vi "RM.getAllDeviceInfo.vi"(8 "error in":errorcluster, 11 "Item Ref in":T2 format="%.0x") -> (0 "error out":errorcluster, 2 "deviceInfo array":T1[](array[typedef]) {"cd node ref" format="%.0x"}, 3 "Item Ref out":T2 format="%.0x")   [LabVIEW 2016, in "FPGA Resource Manager.lvlib"]
uses:
  FPGA Resource Manager.lvlib
  <vilib>/NI Veristand/Custom Device API/Custom Device Item Ref.ctl
  RM.serverInfo.ctl
  RM.Globals.vi
  <vilib>/NI Veristand/Custom Device API/Get Item Property (Variant).vi
  <vilib>/NI Veristand/Custom Device API/Get Item Property (String).vi
  <vilib>/NI Veristand/Custom Device API/Custom Device API.lvlib
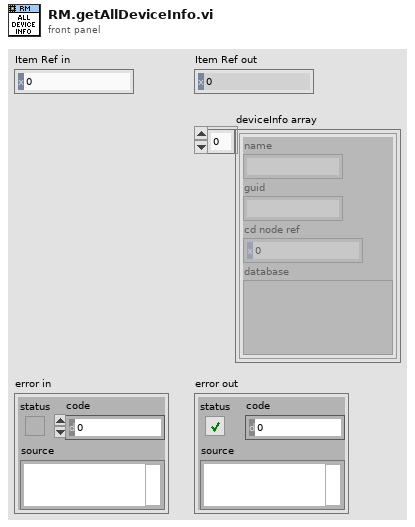
[diagram p1: front panel]
types:
  T1 = typedef "FPGA Resource Manager.lvlib/RM.serverInfo.ctl" = cluster{"name":string, "guid":string, "cd node ref":T2, "database":variant}
  T2 = typedef "Custom Device API.lvlib/Custom Device Item Ref.ctl" = u64
  T3 = typedef "Custom Device API.lvlib/Custom Device Item Info.ctl" = cluster{"Name":string, "Is Channel":bool, "GUID":string, "Is Waveform":bool}
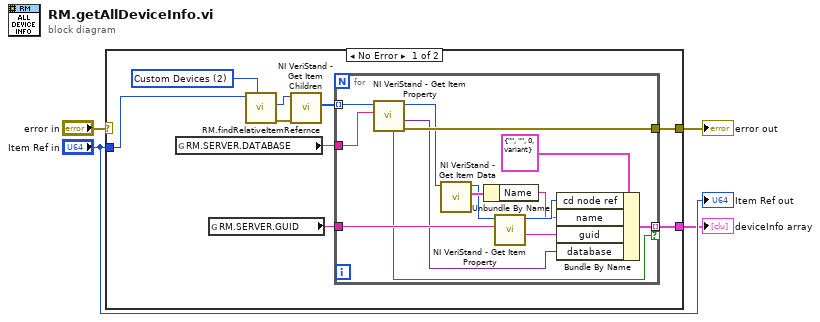
[diagram p0: block diagram]
diagram:
  n1 = case shown="No Error" "error in" {
    selector: "error in" -> [_ w28]
    tunnel: "Item Ref in" -> [w11 _]
    tunnel: [w13 w28] -> w3
    tunnel: [w5 _] -> w1
    frame No Error {
      w12 = u16 2 items=["Targets", "Controller", "Custom Devices", "This CD", "This CD/Group", "This CD/Group/SubGroup"] ("Relative Type")
      n2 = global read "RM.Globals.vi" "RM.SERVER.DATABASE"() -> (w7:string)
      n3 = global read "RM.Globals.vi" "RM.SERVER.GUID"() -> (w6:string)
      n4 = call "RM.findRelativeItemRefernce.vi"("Relative Type"=w12, "Item Ref in"=w11) -> ("error out"=w10:errorcluster, "Relative Item Ref Out"=w9:T2)  [unwired: 5 in, 3 out]
      n5 = call <vilib>:"NI VeriStand - Get Item Children.vi"("error in (no error)"=w10, "Item Ref in"=w9) -> ("Child Refs"=w8:T2[])  [unwired: 6 in, 3 out]
      n6 = for {
        tunnel: w7 -> [w27]
        tunnel: [w26] -> w13
        tunnel: w8 -> [w25] mode=indexing
        tunnel: w6 -> [w21]
        tunnel: [w17] -> w5 mode=indexing if=w20
        n7 = call-poly <vilib>:"NI VeriStand - Get Item Property.vi"("Property Name"=w27, "Item Ref in"=w25) -> ("error out"=w26:errorcluster, "Value"=w14:variant, "Item Ref out"=w24:T2, "Found?"=w20:bool)  [unwired: 6 in]
        n8 = call <vilib>:"NI VeriStand - Get Item Data.vi"("Item Ref in"=w24) -> ("Item Info"=w23:T3, "Item Ref out"=w22:T2)  [unwired: 7 in, 2 out]
        n9 = Unbundle By Name(w23) -> ("Name"=w16:string)
        n10 = call-poly <vilib>:"NI VeriStand - Get Item Property.vi"("Property Name"=w21, "Item Ref in"=w22) -> ("Value"=w15:string, "Item Ref out"=w18:T2)  [unwired: 6 in, 2 out]
        n11 = Bundle By Name(cluster=T1 {"name"="", "guid"="", "cd node ref"=0, "database"=variant} ("deviceInfo"), "cd node ref"=w18, "name"=w16, "guid"=w15, "database"=w14) -> (w17:T1)
      }
    }
    frame Error {
    }
  }
  "error out" <- w3
  "deviceInfo array" <- w1
  "Item Ref out" <- "Item Ref in"
